vi "Write Overlays.vi"(8 "error in (no error)":errorcluster, 10 "Overlays":refnum<class "Shape.lvclass">[](array[class]), 11 "Layered Shape in":refnum<class "Layered Shape.lvclass">) -> (0 "error out":errorcluster, 3 "Layered Shape out":refnum<class "Layered Shape.lvclass">)   [LabVIEW 2015, in "LV Image Editor Framework.lvlib" / "Layered Shape.lvclass"]
uses:
  Layered Shape.lvclass
  Shape/Shape.lvclass
  Layered Shape.lvclass/Layered Shape.ctl
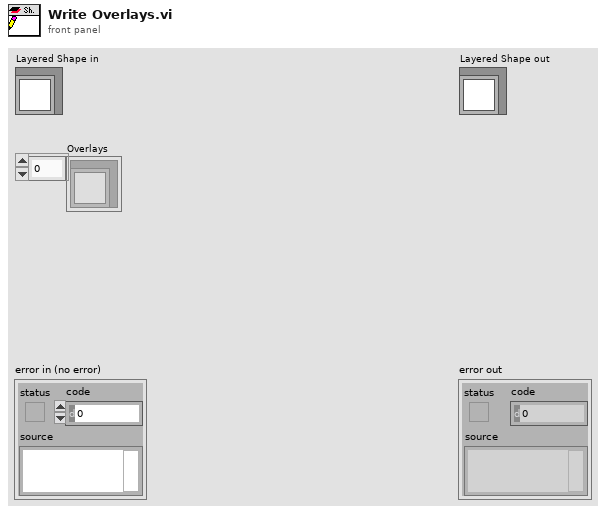
[diagram p1: front panel]
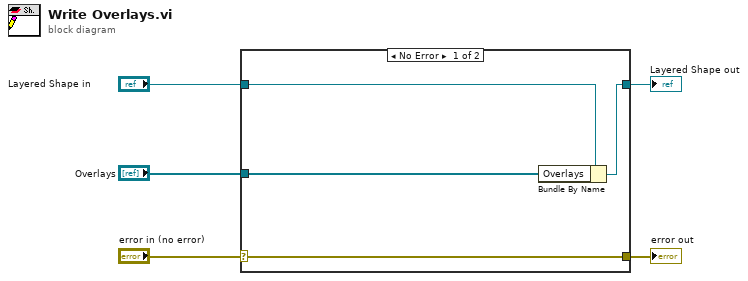
[diagram p0: block diagram]
diagram:
  n1 = case shown="No Error" "error in (no error)" {
    selector: "error in (no error)" -> [w9 w10]
    tunnel: [w9 w10] -> w4
    tunnel: [w7 w11] -> w2
    tunnel: "Layered Shape in" -> [w8 w11]
    tunnel: "Overlays" -> [w6 _]
    frame No Error {
      n2 = Bundle By Name(cluster=w8, "Overlays"=w6) -> (w7:refnum<class "Layered Shape.lvclass">)
    }
    frame Error {
    }
  }
  "error out" <- w4
  "Layered Shape out" <- w2
